vi "INIT DAQs.vi"(8 "error in (no error)":errorcluster, 11 "GlobalData":T1) -> (0 "error out":errorcluster, 3 "Pressure":refnum<k21>)   [LabVIEW 2024]
doc: "Initialize cDAQ to start acquisition data"
uses:
  controls/GlobalData.ctl
  controls/GlobalData.vi
  <vilib>/DAQmx/create/channels.llb/DAQmx Create Channel (AI-Voltage-Basic).vi
  <vilib>/DAQmx/create/channels.llb/DAQmx Create Channel (AI-Current-Basic).vi
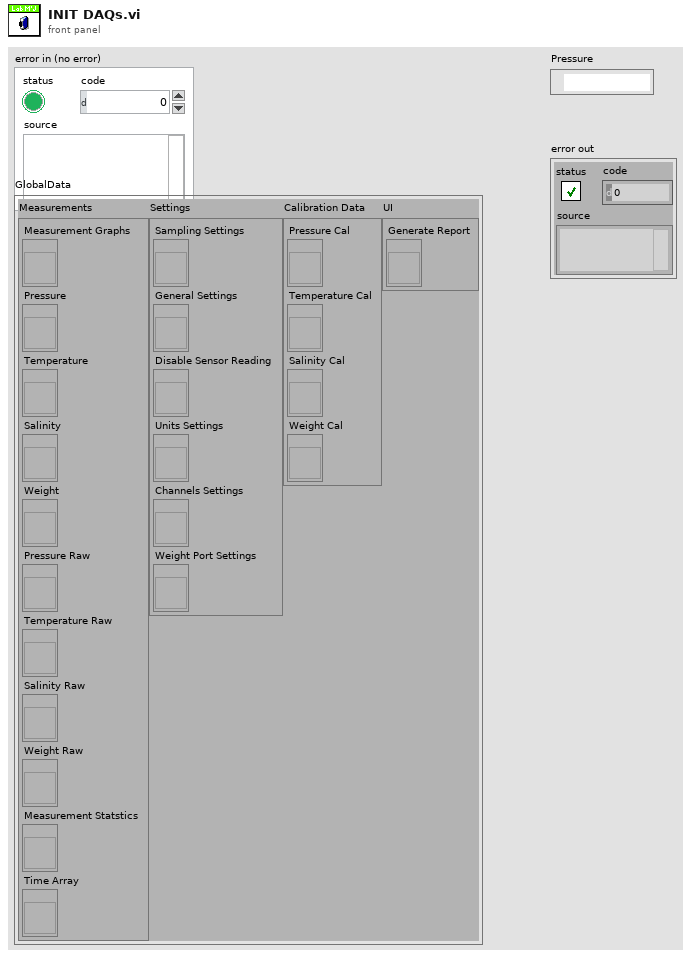
[diagram p1: front panel]
types:
  T1 = typedef "GlobalData.ctl" = cluster{"Measurements":cluster{"Measurement Graphs":refnum<vi>, "Pressure":refnum<vi>, "Temperature":refnum<vi>, "Salinity":refnum<vi>, "Weight":refnum<vi>, "Pressure Raw":refnum<vi>, "Temperature Raw":refnum<vi>, "Salinity Raw":refnum<vi>, "Weight Raw":refnum<vi>, "Measurement Statstics":refnum<vi>, "Time Array":refnum<vi>}, "Settings":cluster{"Sampling Settings":refnum<vi>, "General Settings":refnum<vi>, "Disable Sensor Reading":refnum<vi>, "Units Settings":refnum<vi>, "Channels Settings":refnum<vi>, "Weight Port Settings":refnum<vi>}, "Calibration Data":cluster{"Pressure Cal":refnum<vi>, "Temperature Cal":refnum<vi>, "Salinity Cal":refnum<vi>, "Weight Cal":refnum<vi>}, "UI":cluster{"Generate Report":refnum<vi>}}
  T2 = cluster{"Pressure":cluster{"Physical Channel":tag, "Min Voltage":dbl, "Max Voltage ":dbl, "Terminal Configuration":i32}, "Temperature":cluster{"Physical Channel":tag, "Min Current (mA)":dbl, "Max Current (mA)":dbl, "Terminal Configuration":i32}, "Sallinity":cluster{"Physical Channel":tag, "Min Current (mA)":dbl, "Max Current (mA)":dbl, "Terminal Configuration":i32}}
  T3 = cluster{"Physical Channel":tag, "Min Current (mA)":dbl, "Max Current (mA)":dbl, "Terminal Configuration":i32}
  T4 = cluster{"Physical Channel":tag, "Min Voltage":dbl, "Max Voltage ":dbl, "Terminal Configuration":i32}
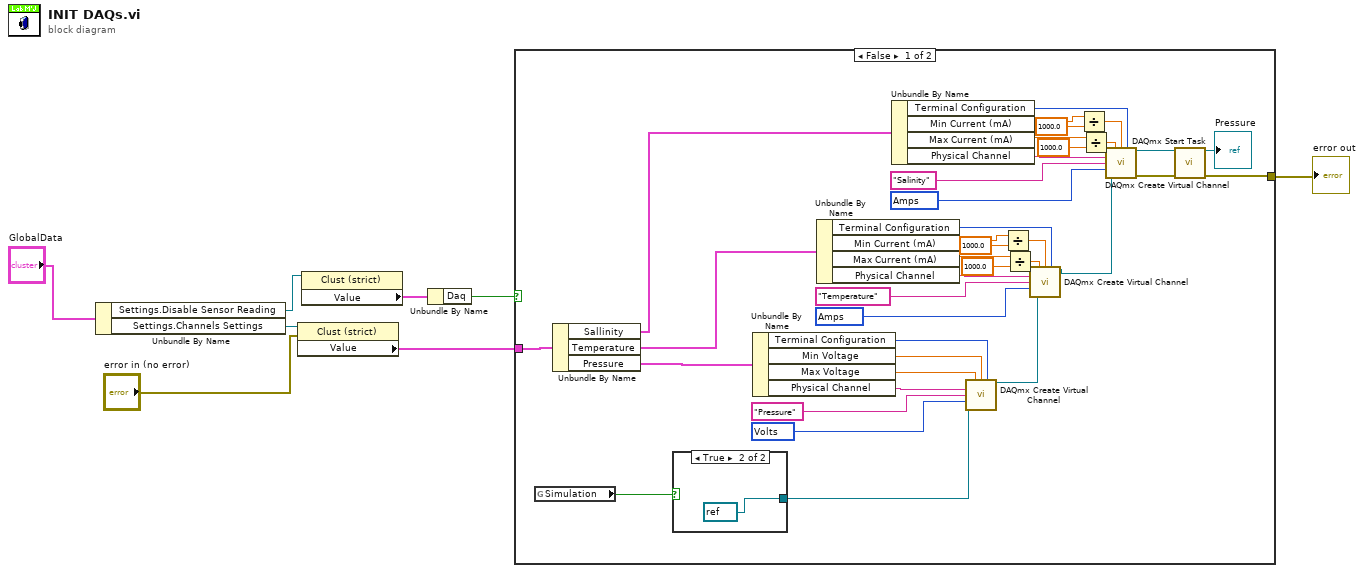
[diagram p0: block diagram]
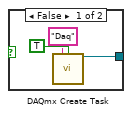
[diagram p2: hidden frame]
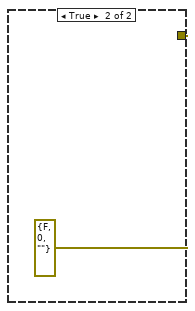
[diagram p3: hidden frame]
diagram:
  n1 = Unbundle By Name("GlobalData") -> ("Settings.Disable Sensor Reading"=w3:refnum<vi>, "Settings.Channels Settings"=w8:refnum<vi>)
  n2 = property class="Clust (strict)"(reference=w8, error in="error in (no error)") -> ("Value"=w7:T2)  [unwired: 2 out]
  n3 = property class="Clust (strict)"(reference=w3) -> ("Value"=w2:cluster{"Daq":bool, "RS232":bool})  [unwired: 1 in, 2 out]
  n4 = Unbundle By Name(w2) -> ("Daq"=w1:bool)
  n5 = case shown="False" w1 {
    tunnel: w7 -> [w26 _]
    tunnel: [w46 errorcluster {"status"=FALSE, "code"=0, "source"=""} ("error out")] -> w6
    frame False {
      w10 = 10342 items=["Amps"=10342, "From Custom Scale"=10065] ("units")
      w11 = 10342 items=["Amps"=10342, "From Custom Scale"=10065] ("units")
      w30 = 10348 items=["Volts"=10348, "From Custom Scale"=10065] ("units")
      n6 = global read "GlobalData.vi" "Simulation"() -> (w45:bool)
      n7 = Unbundle By Name(w26) -> ("Sallinity"=w16:T3, "Temperature"=w25:T3, "Pressure"=w43:T4)
      n8 = case shown="True" w45 {
        tunnel: [w49 refnum<k21> refnum ("task out")] -> w44
        frame False {
          n9 = call <vilib>:"DAQmx Create Task.vi"("new task name"="Daq" ("name to assign"), "auto cleanup"=TRUE) -> ("task out"=w49:refnum<k21>)  [unwired: 12 in, 1 out]
        }
        frame True {
        }
      }
      n10 = Unbundle By Name(w43) -> ("Terminal Configuration"=w42:i32, "Min Voltage"=w29:dbl, "Max Voltage"=w28:dbl, "Physical Channel"=w41:tag)
      n11 = Unbundle By Name(w25) -> ("Terminal Configuration"=w32:i32, "Min Current (mA)"=w34:dbl, "Max Current (mA)"=w38:dbl, "Physical Channel"=w33:tag)
      n12 = Unbundle By Name(w16) -> ("Terminal Configuration"=w24:i32, "Min Current (mA)"=w22:dbl, "Max Current (mA)"=w18:dbl, "Physical Channel"=w23:tag)
      n13 = call-poly <vilib>:"DAQmx Create Virtual Channel.vi"("task in"=w44, "maximum value"=w28, "minimum value"=w29, "input terminal configuration"=w42, "physical channels"=w41, "name to assign"="Pressure", "units"=w30) -> ("task out"=w27:refnum<k21>)  [unwired: 7 in, 1 out]
      n14 = Divide(x=w34, y=1000.0) -> (x/y=w36:dbl)
      n15 = Divide(x=w38, y=1000.0) -> (x/y=w39:dbl)
      n16 = call-poly <vilib>:"DAQmx Create Virtual Channel.vi"("task in"=w27, "maximum value"=w39, "minimum value"=w36, "input terminal configuration"=w32, "physical channels"=w33, "name to assign"="Temperature", "units"=w11) -> ("task out"=w15:refnum<k21>)  [unwired: 7 in, 1 out]
      n17 = Divide(x=w22, y=1000.0) -> (x/y=w20:dbl)
      n18 = Divide(x=w18, y=1000.0) -> (x/y=w17:dbl)
      n19 = call-poly <vilib>:"DAQmx Create Virtual Channel.vi"("task in"=w15, "maximum value"=w17, "minimum value"=w20, "input terminal configuration"=w24, "physical channels"=w23, "name to assign"="Salinity", "units"=w10) -> ("task out"=w13:refnum<k21>, "error out"=w14:errorcluster)  [unwired: 7 in]
      n20 = call <vilib>:"DAQmx Start Task.vi"("task/channels in"=w13, "error in"=w14) -> ("task out"=→"Pressure":refnum<k21>, "error out"=w46:errorcluster)  [unwired: 12 in]
    }
    frame True {
    }
  }
  "error out" <- w6
